vi "GetUpdateEvent.vi"(8 "error in (no error)":errorcluster, 11 "VariableManagerRef in":refnum<vi>) -> (0 "error out":errorcluster, 2 "UpdateEvent":refnum<user-event>, 3 "VariableManagerRef out":refnum<vi>)   [LabVIEW 2013, in "VariableManagerAPI.lvlib"]
doc: "Return the update event of VariableManager object.\n\nUpdate event string list:\n\nVariables\nSequenceIndices\nVariableGroups\nUpdateEvent\nSequenceValues\nLastAcquireValues\nStopUI"
uses:
  VariableManagerAPI.lvlib
  VariableManager/VariableManager.lvclass
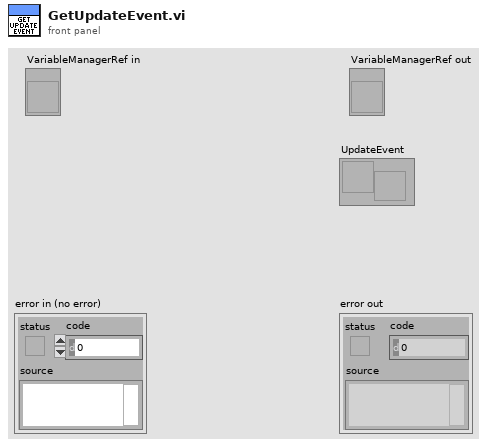
[diagram p1: front panel]
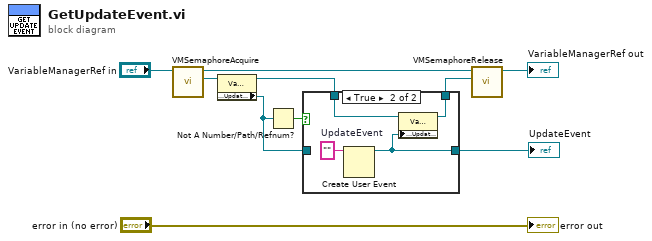
[diagram p0: block diagram]
diagram:
  n1 = call "VMSemaphoreAcquire.vi"("VariableManagerRef in"="VariableManagerRef in") -> ("VariableManager"=w7:refnum<class "VariableManager.lvclass">, "VariableManagerRef out"=w9:refnum<vi>)  [unwired: 7 in, 2 out]
  n2 = property class="VariableManager.lvclass"(reference=w7) -> (reference out=w2:refnum<class "VariableManager.lvclass">, "Accessors:UpdateEvent"=w4:refnum<user-event>)  [unwired: 1 in, 1 out]
  n3 = Not A Number/Path/Refnum?(number/path/refnum=w4) -> (NaN/Path/Refnum?=w5:bool)
  n4 = case shown="True" w5 {
    tunnel: [w12 w15] -> w3
    tunnel: w4 -> [w12 _]
    tunnel: w2 -> [w11 w14]
    tunnel: [w11 w13] -> w1
    frame False {
    }
    frame True {
      w16 = ""  # UpdateEvent
      n5 = Create User Event(user event datatype=w16) -> (user event=w15:refnum<user-event>)  [unwired: 1 in, 1 out]
      n6 = property class="VariableManager.lvclass"(reference=w14, "Accessors:UpdateEvent"=w15) -> (reference out=w13:refnum<class "VariableManager.lvclass">)  [unwired: 1 in, 1 out]
    }
  }
  "UpdateEvent" <- w3
  n7 = call "VMSemaphoreRelease.vi"("VariableManager"=w1, "VariableManagerRef in"=w9) -> ("VariableManagerRef out"=→"VariableManagerRef out":refnum<vi>)  [unwired: 8 in, 1 out]
  "error out" <- "error in (no error)"
